vi "CAN.vi"() -> (1 "CAN Sele":T1=enum."TFT/LCD Power Off", 2 "CAN":bool, 3 "Out":bool)   [LabVIEW 2015]
uses:
  Control Button/Exit.ctl
  Control PB/Next_.ctl
  Control PB/CAN.ctl
panel:
  in  "CAN Selection":T1=enum."TFT/LCD Power Off"
  in  "Barcode":bool
  in  "Next":T2
  in  "Exit":T3
  # "Add Feature List"
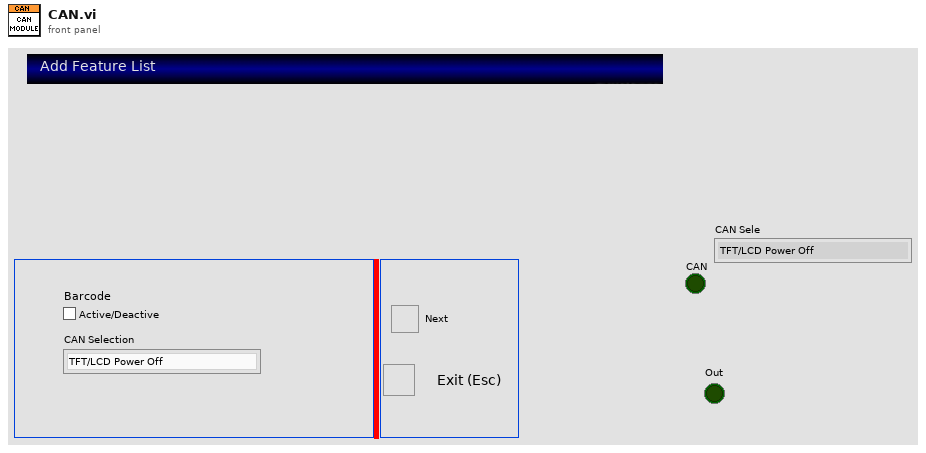
[diagram p1: front panel]
types:
  T1 = typedef "CAN.ctl" = enum16{"TFT/LCD Power On", "TFT/LCD Power Off", "KM CHeck"}
  T2 = typedef "Next_.ctl" = bool
  T3 = typedef "Exit.ctl" = bool
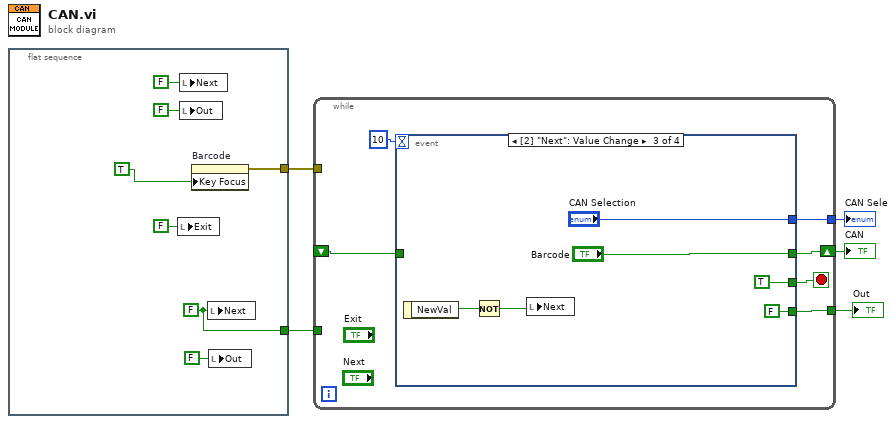
[diagram p0: block diagram]
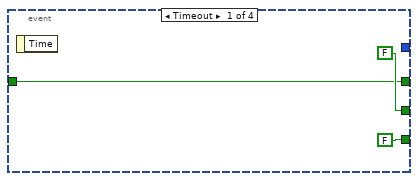
[diagram p2: hidden frame]
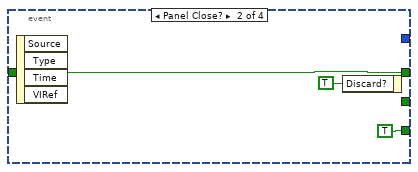
[diagram p3: hidden frame]
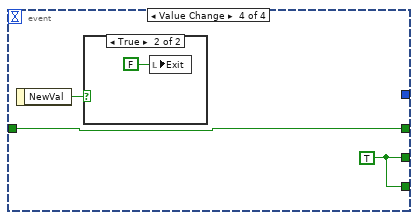
[diagram p4: hidden frame]
diagram:
  n1 = flat-sequence {
    tunnel: [w9] -> w4
    tunnel: [w6] -> w3
    frame #0 {
      w9 = T2 FALSE ("Next")
      n2 = local write "Exit"(FALSE ("Exit")) -> ()
      n3 = local write "Next"(T2 FALSE ("Next")) -> ()
      n4 = local write "Out"(FALSE ("Out")) -> ()
      n5 = property on="Barcode" class="Bool (strict)"("Key Focus"=TRUE) -> (error out=w6:errorcluster)  [unwired: 2 in, 1 out]
      n6 = local write "Next"(w9) -> ()
      n7 = local write "Out"(FALSE ("Out")) -> ()
    }
  }
  n8 = while {
    tunnel: [w16] -> w5
    tunnel: w4 -> [_]
    shift-right: [w17] -> w2
    shift-left: _ -> [w14]
    tunnel: w3 -> [_]
    tunnel: [w13] -> w1
    stop <- w18 stop-if-true
    n9 = event shown="[2] \"Next\": Value Change" {
      selector: _ -> [_ _ _ _]
      dyn-events: _ -> [_ _ _ _]
      timeout: 10 -> [_ _ _ _]
      tunnel: [FALSE _ T2 TRUE ("NewVal") w31] -> w18
      tunnel: [w19 w22 "Barcode" w32] -> w17
      tunnel: [T2 FALSE ("NewVal") T2 TRUE ("NewVal") T2 FALSE ("NewVal") w31] -> w16
      tunnel: w14 -> [w19 w22 _ w32]
      tunnel: [_ _ "CAN Selection" _] -> w13
      event Timeout {
        n10 = event-data() -> ()  [unwired: 1 in, 1 out]
      }
      event Panel Close? {
        n11 = event-data() -> ()  [unwired: 1 in, 4 out]
        n12 = event-data("Discard?"=TRUE) -> ()  [unwired: 1 in, 1 out]
      }
      event Value Change {
        n13 = event-data() -> ("NewVal"=w27:T2)  [unwired: 1 in]
        n14 = Not(x=w27) -> (.not. x?=w26:T2)
        n15 = local write "Next"(w26) -> ()
      }
      event Value Change {
        w31 = TRUE
        n16 = event-data() -> ("NewVal"=w33:T3)  [unwired: 1 in]
        n17 = case shown="True" w33 {
          frame False {
          }
          frame True {
            n18 = local write "Exit"(T2 FALSE ("Next")) -> ()
          }
        }
      }
    }
  }
  "Out" <- w5
  "CAN" <- w2
  "CAN Sele" <- w1
